vi "Untitled 18 (SubVI).vi"(8 "Cpair":dbl, 10 "Numeric in":dbl, 11 "Compressor inlet Tempreture (K)":dbl) -> (3 "Numeric out":dbl)   [LabVIEW 2019]
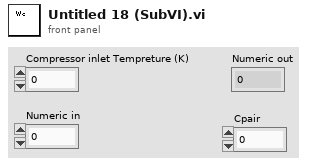
[diagram p1: front panel]
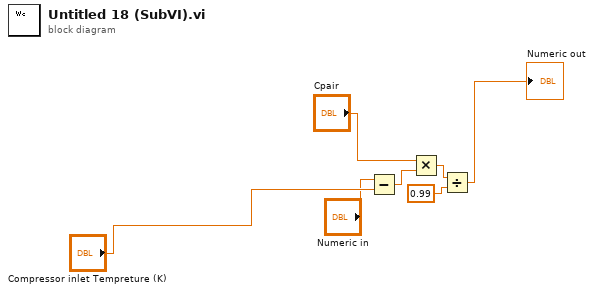
[diagram p0: block diagram]
diagram:
  n1 = Subtract(x="Numeric in", y="Compressor inlet Tempreture (K)") -> (x-y=w4:dbl)
  n2 = Multiply(x="Cpair", y=w4) -> (x*y=w5:dbl)
  n3 = Divide(x=w5, y=0.99) -> (x/y=→"Numeric out":dbl)
